vi "Read FPGA Ref.vi"(8 "error in (no error)":errorcluster, 11 "FPGA Vaisala in":refnum<class "FPGA Vaisala.lvclass">) -> (0 "error out":errorcluster, 2 "FPGA Ref":refnum<k20>, 3 "FPGA Vaisala out":refnum<class "FPGA Vaisala.lvclass">)   [LabVIEW 2014, in "FPGA Vaisala.lvclass"]
uses:
  FPGA Vaisala.lvclass
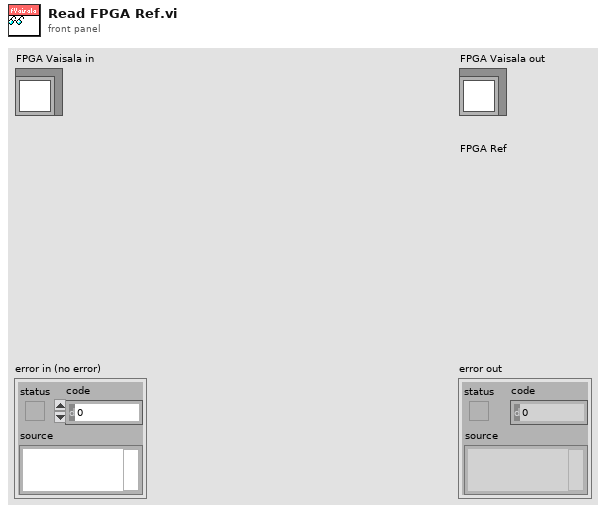
[diagram p1: front panel]
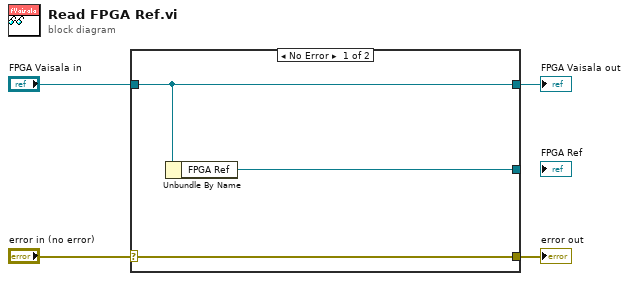
[diagram p0: block diagram]
diagram:
  n1 = case shown="No Error" "error in (no error)" {
    selector: "error in (no error)" -> [w7 w8]
    tunnel: [w7 w8] -> w3
    tunnel: [w6 w9] -> w1
    tunnel: "FPGA Vaisala in" -> [w6 w9]
    tunnel: [w5 _] -> _
    frame No Error {
      n2 = Unbundle By Name(w6) -> ("FPGA Ref"=w5:refnum<k20>)
    }
    frame Error {
    }
  }
  "error out" <- w3
  "FPGA Vaisala out" <- w1
